vi "SQL_Table_Test_Insert.vi"(8 "试验开始日期":string, 11 "用户名":string) -> (3 "error out":errorcluster)   [LabVIEW 2014]
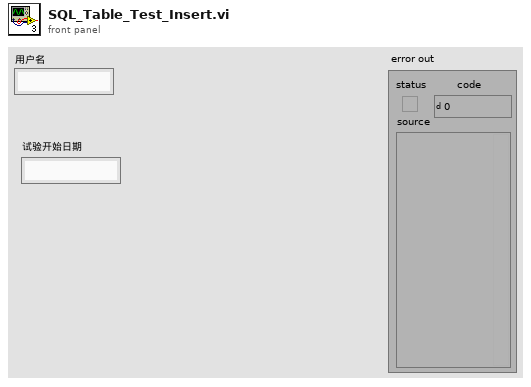
[diagram p1: front panel]
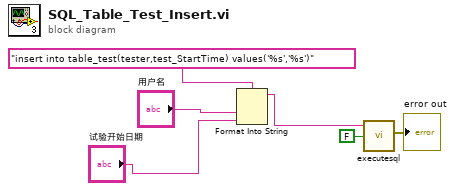
[diagram p0: block diagram]
diagram:
  n1 = Format Into String(format string="insert into table_test(tester,test_StartTime) values('%s','%s')" ("Command Text"), "用户名", "试验开始日期") -> (resulting string=w4:string)  [unwired: 2 in, 1 out]
  n2 = call "executesql.vi"("Return Data (T)"=FALSE, "Command Text"=w4) -> ("error out"=→"error out":errorcluster)  [unwired: 5 in, 1 out]
